vi "Temp_Splitter_DAQ1_SUBVI.vi"(10 "DAQ_OUT":dbl[](array[numeric]), 11 "Tomt Array":dbl[](array[numeric])) -> (0 "Counter_Array":dbl[](array[numeric]), 1 "TEMP3":dbl[](array[numeric]), 2 "TEMP2":dbl[](array[numeric]), 3 "TEMP1":dbl[](array[numeric]))   [LabVIEW 2022 SP3]
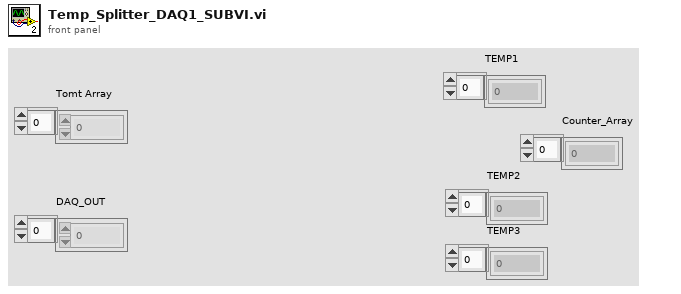
[diagram p1: front panel]
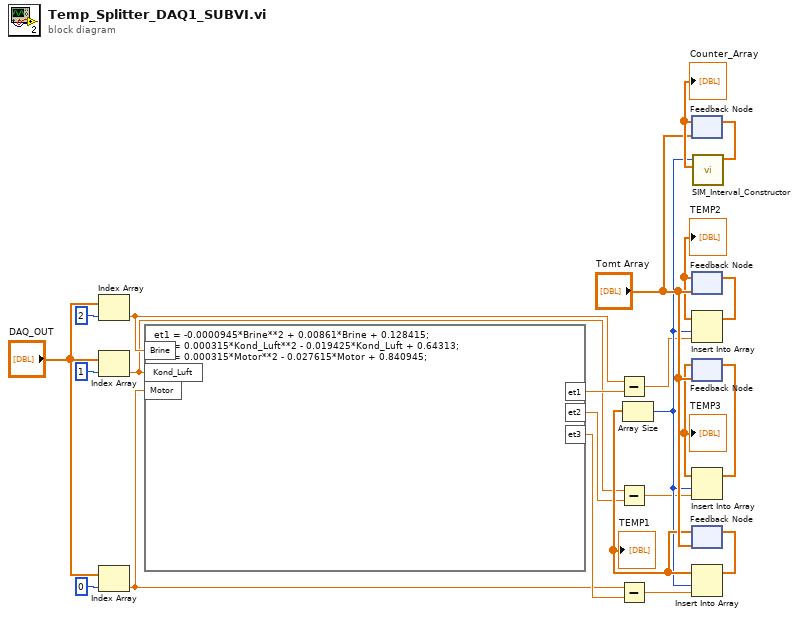
[diagram p0: block diagram]
diagram:
  n1 = Index Array(array="DAQ_OUT", index=2) -> (element=w6:dbl)
  n2 = Index Array(array="DAQ_OUT", index=1) -> (element=w4:dbl)
  n3 = Index Array(array="DAQ_OUT", index=0) -> (element=w2:dbl)
  n4 = formula code="et1 = -0.0000945*Brine**2 + 0.00861*Brine + 0.128415;\net2 = 0.000315*Kond_Luft**2 - 0.019425*Kond_Luft + 0.64313;\net3 = 0.000315*Motor**2 - 0.027615*Motor + 0.840945;"("Brine"=w6, "Kond_Luft"=w4, "Motor"=w2) -> ("et1"=w9:dbl, "et2"=w8:dbl, "et3"=w7:dbl)
  n5 = Subtract(x=w6, y=w9) -> (x-y=w5:dbl)
  n6 = Subtract(x=w4, y=w8) -> (x-y=w3:dbl)
  n7 = Subtract(x=w2, y=w7) -> (x-y=w1:dbl)
  n8 = feedback #1("Tomt Array") -> (w23:dbl[])
  "Counter_Array" <- w23
  n9 = feedback #2("Tomt Array") -> (w20:dbl[])
  "TEMP2" <- w20
  n10 = feedback #3("Tomt Array") -> (w18:dbl[])
  "TEMP3" <- w18
  n11 = feedback #4("Tomt Array") -> (w16:dbl[])
  "TEMP1" <- w16
  n12 = Array Size(array=w16) -> (size(s)=w14:i32)
  n13 = Insert Into Array(array=w20, index=w14, new element=w5) -> (w19:dbl[])
  n14 = feedback-in #2(w19) -> ()
  n15 = Insert Into Array(array=w18, index=w14, new element=w3) -> (w17:dbl[])
  n16 = feedback-in #3(w17) -> ()
  n17 = Insert Into Array(array=w16, index=w14, new element=w1) -> (w15:dbl[])
  n18 = feedback-in #4(w15) -> ()
  n19 = call "SIM_Interval_Constructor.vi"("History Data in"=w23, "size(s)"=w14) -> ("History Data out"=w22:dbl[])  [unwired: 9 in]
  n20 = feedback-in #1(w22) -> ()
